vi "MoveTime.vi"(1 "maxaccel":dbl=3.0 min=1e-50 max=1e+50, 2 "maxspeed":dbl=2.0, 3 "dist":dbl=1.0) -> (0 "expected duration":dbl=1.1547005383792515)   [LabVIEW 2011]
panel:
  out "2accelDist":dbl=1.3333333333333333
  # "use the same dimmensions!\nm;m/s;m/s^2\nmm;mm/s;mm/s^2"
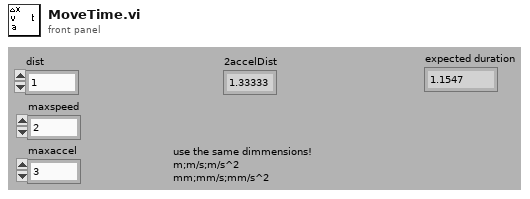
[diagram p1: front panel]
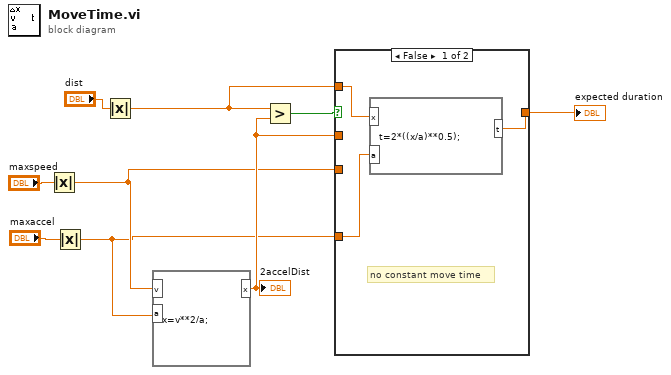
[diagram p0: block diagram]
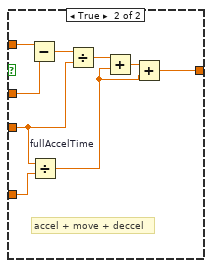
[diagram p2: hidden frame]
diagram:
  n1 = Absolute Value(x="maxspeed") -> (abs(x)=w3:dbl)
  n2 = Absolute Value(x="maxaccel") -> (abs(x)=w2:dbl)
  n3 = Absolute Value(x="dist") -> (abs(x)=w1:dbl)
  n4 = formula code="x=v**2/a;"("v"=w3, "a"=w2) -> ("x"=w7:dbl)
  "2accelDist" <- w7
  n5 = Greater?(x=w1, y=w7) -> (0:w9:bool)
  n6 = case shown="False" w9 {
    tunnel: w1 -> [w12 w21]
    tunnel: w7 -> [_ w20]
    tunnel: w3 -> [_ w15]
    tunnel: [w11 w16] -> w5
    tunnel: w2 -> [w10 w14]
    frame False {
      # "no constant move time"
      n7 = formula code="t=2*((x/a)**0.5);"("x"=w12, "a"=w10) -> ("t"=w11:dbl)
    }
    frame True {
      # "accel + move + deccel"
      n8 = Subtract(x=w21, y=w20) -> (x-y=w19:dbl)
      n9 = Divide "fullAccelTime"(x=w15, y=w14) -> (x/y=w13:dbl)
      n10 = Divide(x=w19, y=w15) -> (x/y=w18:dbl)
      n11 = Add(x=w18, y=w13) -> (x+y=w17:dbl)
      n12 = Add(x=w17, y=w13) -> (x+y=w16:dbl)
    }
  }
  "expected duration" <- w5
